vi "SAHarmonicDistortionRangeTableConfigureFrequency.vi"(8 "error in (no error)":errorcluster {"code" format="%.0x"}, 9 "Frequency":dbl[](array[numeric])=[0.0, 0.0, 0.0, 0.0, 0.0, 0.0, 0.0, 0.0, 0.0, 0.0] format="%.2p", 11 "instrument handle":refnum<k15>) -> (0 "error out":errorcluster {"code" format="%.0x"}, 3 "instrument handle out":refnum<k15>)   [LabVIEW 2009, in "Keysight XSAn.lvlib"]
doc: "Sets the frequency of the harmonics.\n\nSupported Models: M9290A, N8973B, N8974B, N8975B, N8976B, N9000A, N9000B, N9010A, N9010B, N9020A, N9020B, N9030A, N9030B, N9038A, N9040B, N9041B, SPN9003A, SPN9026A"
uses:
  <instrlib>/Keysight XSAn/Keysight XSAn.lvlib
  AgXSAn.dll
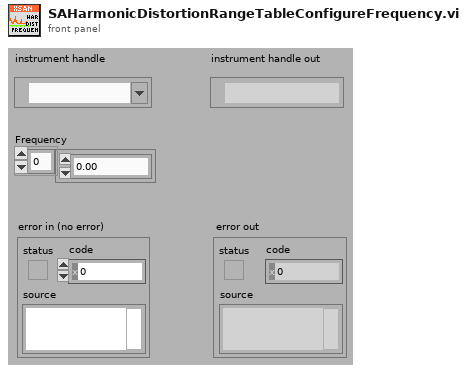
[diagram p1: front panel]
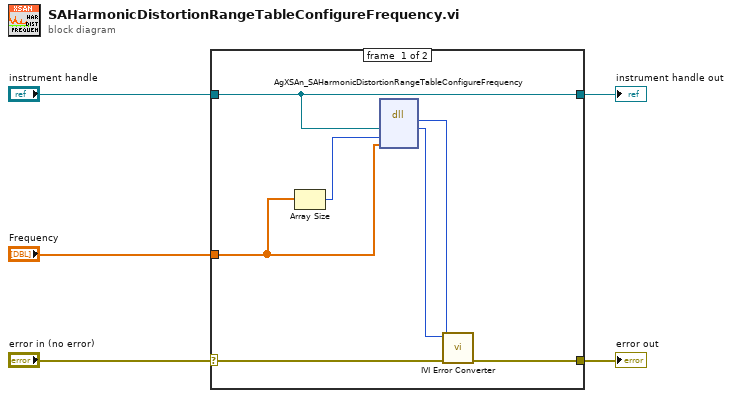
[diagram p0: block diagram]
diagram:
  n1 = case shown="No Error" "error in (no error)" {
    selector: "error in (no error)" -> [w10 w14]
    tunnel: [w9 w14] -> w5
    tunnel: "instrument handle" -> [w8 w13]
    tunnel: "Frequency" -> [w7 _]
    tunnel: [w8 w13] -> w1
    frame #0 {
      n2 = Array Size(array=w7) -> (size(s)=w6:i32)
      n3 = dll-call lib="AgXSAn**.dll" fn="AgXSAn_SAHarmonicDistortionRangeTableConfigureFrequency"("Vi"=w8, "FrequencyBufferSize"=w6, "Frequency"=w7) -> (w11:i32, "Vi"=w12:u32)  [unwired: 5 in, 2 out]
      n4 = call <instrlib>:"IVI Error Converter.vi"("error in (no error)"=w10, "IVI error code (0)"=w11, "instrument handle"=w12) -> ("error out"=w9:errorcluster)  [unwired: 7 in, 1 out]
    }
    frame #1 {
    }
  }
  "error out" <- w5
  "instrument handle out" <- w1
